vi "Note Result.vi"(8 "error in (no error)":errorcluster, 9 "Stage":enum16{"Init", "Work"}(ring), 10 "Acquired Result.lvclass":refnum<class "Acquired Result.lvclass">, 11 "Measure Controller in":refnum<class "Process Controller.lvclass">) -> (0 "error out":errorcluster, 3 "Measure Controller out":refnum<class "Process Controller.lvclass">)   [LabVIEW 2016, in "Process Controller.lvclass"]
uses:
  Process Controller.lvclass
  NHMFL_Core/Libraries/Instruments/Results/Acquired Result/Acquired Result.lvclass
  NHMFL_Core/Libraries/Instruments/Results/Acquired Result/Acquired Result.lvclass/Acquired Result.ctl
  Process Controller.lvclass/Process Controller.ctl
  NHMFL_Core/Libraries/Instruments/Results/Acquired Result/Read Sender.vi
  NHMFL_Core/Libraries/Instruments/Results/Acquired Result/Read Final.vi
  NHMFL_Core/Libraries/Instruments/Results/Acquired Result/Read Cycle count.vi
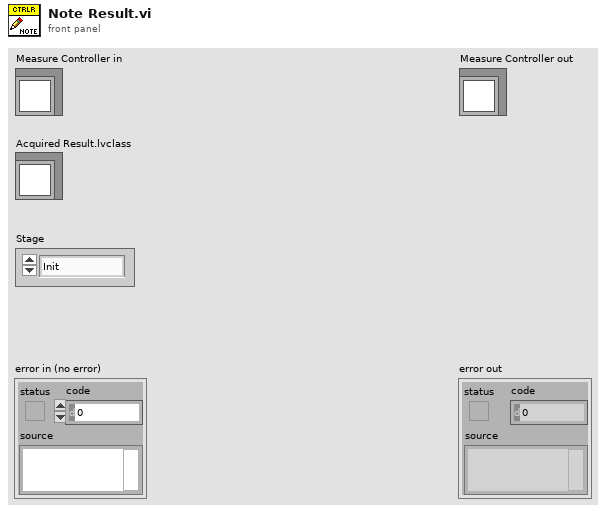
[diagram p1: front panel]
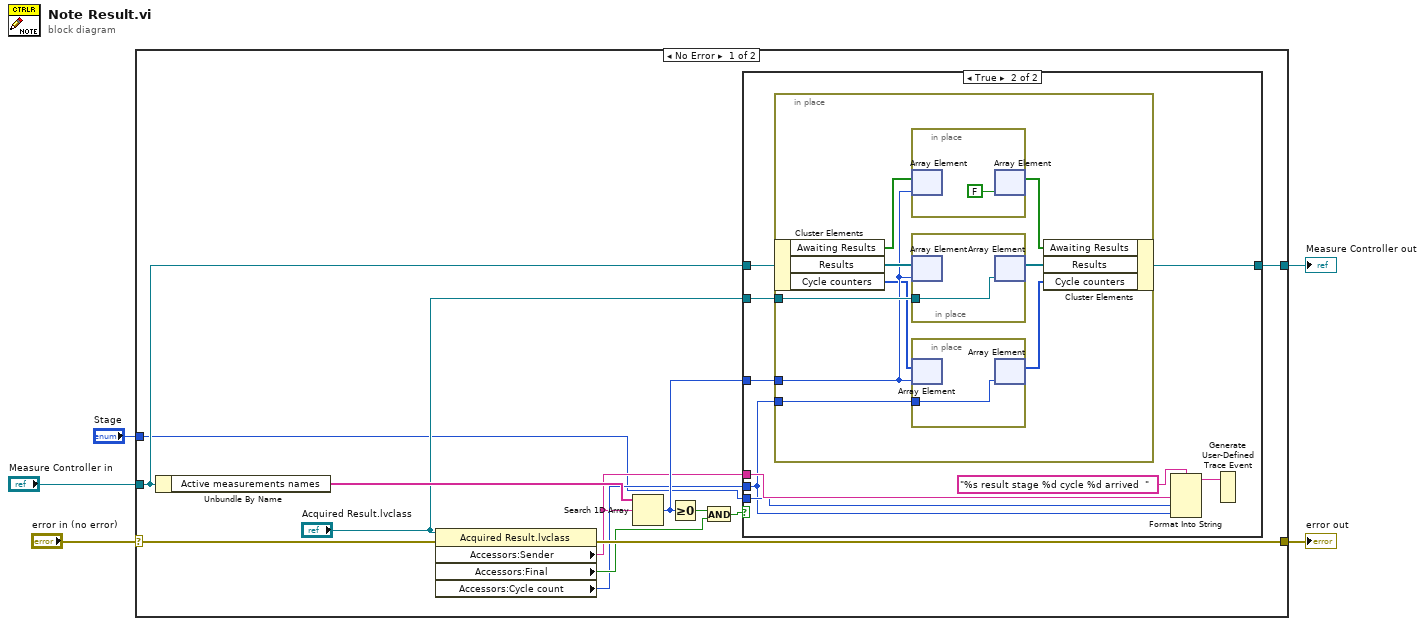
[diagram p0: block diagram]
diagram:
  n1 = case shown="No Error" "error in (no error)" {
    selector: "error in (no error)" -> [w16 w42]
    tunnel: [w15 w42] -> w4
    tunnel: [w13 w41] -> w2
    tunnel: "Measure Controller in" -> [w14 w41]
    tunnel: "Stage" -> [w6 _]
    frame No Error {
      n2 = Unbundle By Name(w14) -> ("Active measurements names"=w18:string[])
      n3 = property class="Acquired Result.lvclass"(reference="Acquired Result.lvclass", error in=w16) -> (error out=w15:errorcluster, "Accessors:Sender"=w7:string, "Accessors:Final"=w9:bool, "Accessors:Cycle count"=w8:i32)  [unwired: 1 out]
      n4 = Search 1D Array(1D array=w18, element=w7) -> (index of element=w11:i32)  [unwired: 1 in]
      n5 = Greater Or Equal To 0?(x=w11) -> (x >= 0?=w12:bool)
      n6 = And(x=w12, y=w9) -> (x .and. y?=w10:bool)
      n7 = case shown="True" w10 {
        tunnel: w11 -> [_ w28]
        tunnel: "Acquired Result.lvclass" -> [_ w27]
        tunnel: w14 -> [w19 w26]
        tunnel: [w19 w25] -> w13
        tunnel: w8 -> [_ w21]
        tunnel: w7 -> [_ w23]
        tunnel: w6 -> [_ w22]
        frame False {
        }
        frame True {
          n8 = in-place {
            in-place-border: w28 -> [w32]
            in-place-border: w27 -> [w34]
            in-place-border: w21 -> [w31]
            n9 = in-place-cluster #1(w26) -> ("Awaiting Results"=w37:bool[], "Results"=w35:refnum<class "Acquired Result.lvclass">[], "Cycle counters"=w30:i32[])
            n10 = in-place {
              n11 = in-place-array #2(w37, w32) -> ()  [unwired: 1 out]
              n12 = in-place-array #2(FALSE ("new element/subarray")) -> (w36:bool[])  [unwired: 1 out]
            }
            n13 = in-place {
              in-place-border: w34 -> [w39]
              n14 = in-place-array #3(w35, w32) -> ()  [unwired: 1 out]
              n15 = in-place-array #3(w39) -> (w33:refnum<class "Acquired Result.lvclass">[])  [unwired: 1 out]
            }
            n16 = in-place {
              in-place-border: w31 -> [w38]
              n17 = in-place-array #4(w30, w32) -> ()  [unwired: 1 out]
              n18 = in-place-array #4(w38) -> (w29:i32[])  [unwired: 1 out]
            }
            n19 = in-place-cluster #1("Awaiting Results"=w36, "Results"=w33, "Cycle counters"=w29) -> (w25:refnum<class "Process Controller.lvclass">)
          }
          n20 = Format Into String(format string="%s result stage %d cycle %d arrived  ", w23, w22, w21) -> (resulting string=w20:string)  [unwired: 2 in, 1 out]
          n21 = Generate User-Defined Trace Event(2:w20) -> ()  [unwired: 1 in]
        }
      }
    }
    frame Error {
    }
  }
  "error out" <- w4
  "Measure Controller out" <- w2
